vi "Aula 5 14_09 Graph_History_FormulaNode.vi"() -> ()   [LabVIEW 2020]
panel:
  out "Ângulo":i32
  out "XY Graph":cluster{i32[], dbl[]}(graph)
  out "Waveform Chart":cluster{"a":dbl, "b":dbl, "c":dbl, "d":dbl}(graph)
  in  "Espera [ms]":u32
  in  "Stop Button":bool
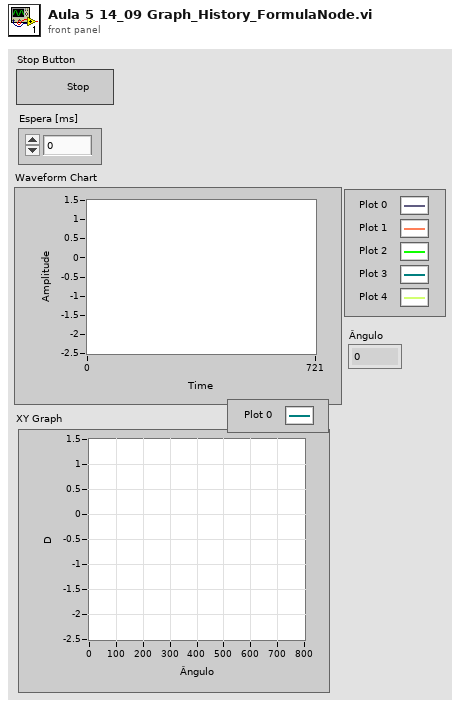
[diagram p1: front panel]
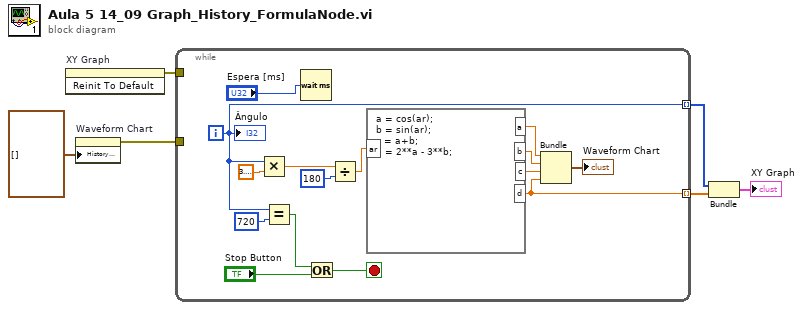
[diagram p0: block diagram]
diagram:
  n1 = invoke on="XY Graph" class="XYGraph (strict)" method="Reinit To Default"() -> (error out=w1:errorcluster)  [unwired: 3 in, 2 out]
  n2 = property on="Waveform Chart" class="WFChart (strict)"("History Data"=cluster{"a":dbl, "b":dbl, "c":dbl, "d":dbl}[] []) -> (error out=w6:errorcluster)  [unwired: 2 in, 1 out]
  n3 = while {
    tunnel: w6 -> [_]
    tunnel: [w12] -> w3 mode=indexing
    tunnel: [w11] -> w4 mode=indexing
    tunnel: w1 -> [_]
    i -> [w11]
    stop <- w7 stop-if-true
    n4 = Multiply(x=w11, y=3.141592653589793) -> (x*y=w19:dbl)
    n5 = Equal?(x=w11, y=720) -> (x = y?=w9:bool)
    n6 = Wait (ms)(milliseconds to wait="Espera [ms]") -> ()  [unwired: 1 out]
    n7 = Or(x=w9, y="Stop Button") -> (x .or. y?=w7:bool)
    n8 = Divide(x=w19, y=180) -> (x/y=w17:dbl)
    n9 = formula code="a = cos(ar);\nb = sin(ar);\nc = a+b;\nd = 2**a - 3**b;"("ar"=w17) -> ("a"=w16:dbl, "b"=w15:dbl, "c"=w14:dbl, "d"=w12:dbl)
    n10 = Bundle("a"=w16, "b"=w15, "c"=w14, "d"=w12) -> (→"Waveform Chart":cluster{"a":dbl, "b":dbl, "c":dbl, "d":dbl})  [unwired: 1 in]
    "Ângulo" <- w11
  }
  n11 = Bundle(w4, w3) -> (→"XY Graph":cluster{i32[], dbl[]})  [unwired: 1 in]
